vi "Recursive Add Item References to Map.vi"(8 "error in (no error)":errorcluster, 10 "ProjectItem Refnum":refnum<vi>, 11 "Icon Decorator In":refnum<class "Icon Decorator.lvclass">) -> (0 "error out":errorcluster, 3 "Icon Decorator Out":refnum<class "Icon Decorator.lvclass">)   [LabVIEW 2020, in "Icon Decorator.lvclass"]
uses:
  Icon Decorator.lvclass
  LUnit Test Case.lvclass
  Icon Decorator.lvclass/Icon Decorator.ctl
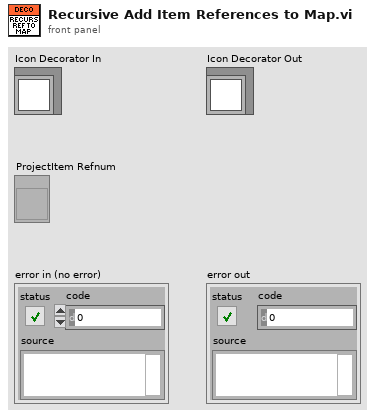
[diagram p1: front panel]
types:
  T1 = typedef "ItemRef.ctl" = u64
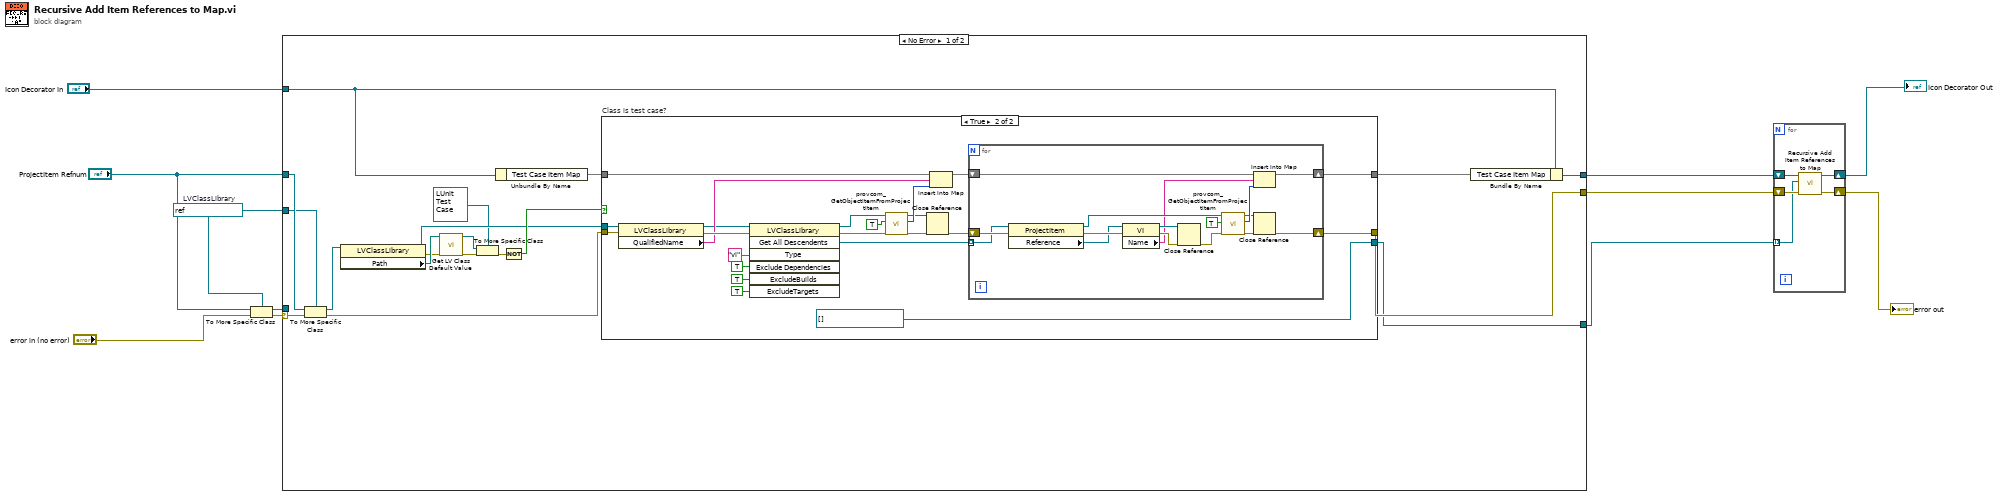
[diagram p0: block diagram]
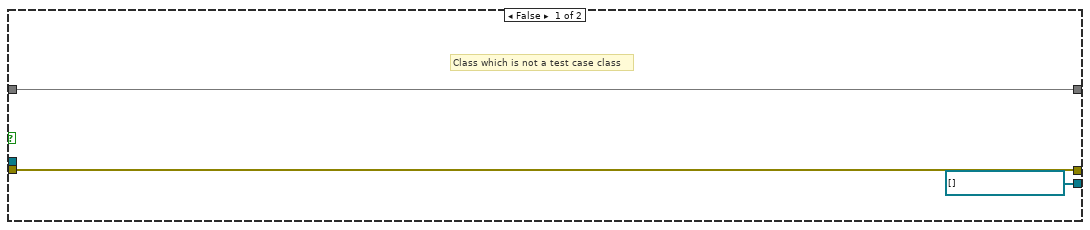
[diagram p2: hidden frame]
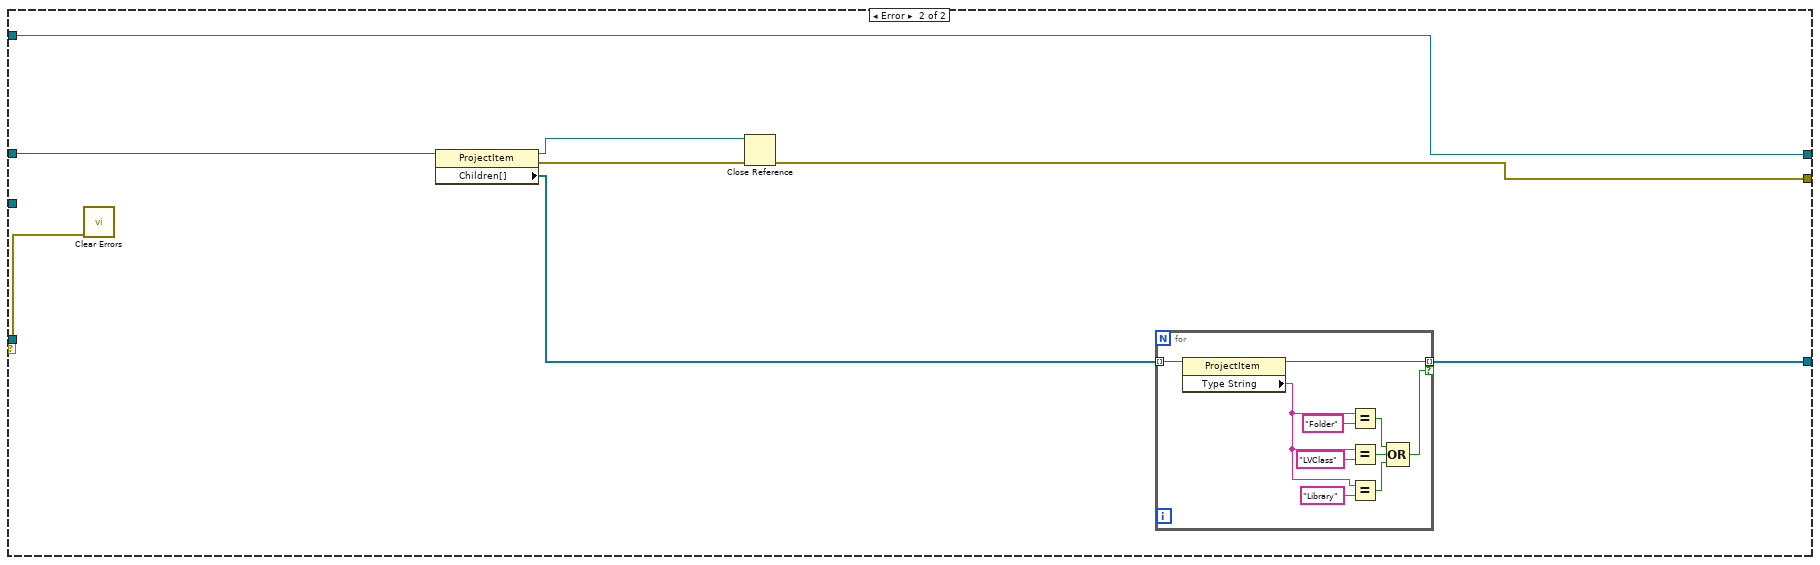
[diagram p3: hidden frame]
diagram:
  w1 = refnum<vi> refnum  # LVClassLibrary
  n1 = To More Specific Class(target class=w1, reference="ProjectItem Refnum", error in="error in (no error)") -> (specific class reference=w3:refnum<vi>, error out=w4:errorcluster)
  n2 = case shown="No Error" w4 {
    selector: w4 -> [w24 w76]
    tunnel: "Icon Decorator In" -> [w30 w74]
    tunnel: [w27 w75] -> w10
    tunnel: [w26 w74] -> w8
    tunnel: [w25 w72] -> w6
    tunnel: w3 -> [_ _]
    tunnel: "ProjectItem Refnum" -> [w22 w77]
    tunnel: w1 -> [w21 _]
    frame No Error {
      n3 = To More Specific Class(target class=w21, reference=w22, error in=w24) -> (specific class reference=w19:refnum<vi>, error out=w23:errorcluster)
      n4 = property class="LVClassLibrary"(reference=w19) -> (reference out=w18:refnum<vi>, error out=w14:errorcluster, "Path"=w15:path)  [unwired: 1 in]
      n5 = call <vilib>:"Get LV Class Default Value.vi"("error in (no error)"=w14, "class path"=w15) -> ("error out"=w12:errorcluster, "object"=w13:refnum<class>)  [unwired: 8 in]
      n6 = To More Specific Class(target class=refnum<class "LUnit Test Case.lvclass"> refnum ("LUnit Test Case V2.lvclass"), reference=w13, error in=w12) -> (error out=w16:errorcluster)  [unwired: 1 out]
      n7 = Unbundle By Name(w30) -> ("Test Case Item Map"=w28:map{string, T1})
      n8 = Not(x=w16) -> (.not. x?=w20:bool)
      n9 = case "Class is test case?" shown="True" w20 {
        tunnel: w28 -> [w33 w54]
        tunnel: w18 -> [_ w53]
        tunnel: w23 -> [w32 w48]
        tunnel: [w32 w38] -> w27
        tunnel: [w33 w40] -> w29
        tunnel: [refnum<vi>[] [] ("Children[]") refnum<vi>[] [] ("Children[]")] -> w25
        frame False {
          # "Class which is not a test case class"
        }
        frame True {
          n10 = property class="LVClassLibrary"(reference=w53, error in=w48) -> (reference out=w43:refnum<vi>, error out=w47:errorcluster, "QualifiedName"=w46:string)
          n11 = invoke class="LVClassLibrary" method="Get All Descendents"(reference=w43, error in=w47, "Type"="vi", "Exclude Dependencies"=TRUE ("ExcludeDependencies"), "ExcludeBuilds"=TRUE, "ExcludeTargets"=TRUE) -> (reference out=w42:refnum<vi>, error out=w44:errorcluster, "All Descendents"=w37:refnum<vi>[])  [unwired: 1 in, 4 out]
          n12 = call <resource>:"provcom_GetObjectItemFromProjectItem.vi"("error in (no error)"=w44, "bind? (Y)"=TRUE, "ProjectItem"=w42) -> ("error out"=w50:errorcluster, "ObjectItem"=w52:T1, "dup ProjectItem"=w51:refnum<vi>)  [unwired: 6 in]
          n13 = Close Reference(reference=w51, error in (no error)=w50) -> (error out=w39:errorcluster)
          n14 = Insert Into Map(map in=w54, key=w46, value=w52) -> (map out=w49:map{string, T1})  [unwired: 2 out]
          n15 = for {
            tunnel: w37 -> [w67] mode=indexing
            shift-right: [w70] -> w40
            shift-left: w49 -> [w71]
            shift-right: [w65] -> w38
            shift-left: w39 -> [w69]
            n16 = property class="ProjectItem"(reference=w67, error in=w69) -> (reference out=w66:refnum<vi>, error out=w68:errorcluster, "Reference"=w64:refnum<vi>)
            n17 = property class="VI"(reference=w64, error in=w68) -> (reference out=w57:refnum<vi>, error out=w59:errorcluster, "Name"=w56:string)
            n18 = Close Reference(reference=w57, error in (no error)=w59) -> (error out=w58:errorcluster)
            n19 = call <resource>:"provcom_GetObjectItemFromProjectItem.vi"("error in (no error)"=w58, "bind? (Y)"=TRUE, "ProjectItem"=w66) -> ("error out"=w62:errorcluster, "ObjectItem"=w63:T1, "dup ProjectItem"=w61:refnum<vi>)  [unwired: 6 in]
            n20 = Insert Into Map(map in=w71, key=w56, value=w63) -> (map out=w70:map{string, T1})  [unwired: 2 out]
            n21 = Close Reference(reference=w61, error in (no error)=w62) -> (error out=w65:errorcluster)
          }
        }
      }
      n22 = Bundle By Name(cluster=w30, "Test Case Item Map"=w29) -> (w26:refnum<class "Icon Decorator.lvclass">)
    }
    frame Error {
      n23 = call <vilib>:"Clear Errors.vi"("error in (no error)"=w76) -> ()  [unwired: 5 in, 2 out]
      n24 = property class="ProjectItem"(reference=w77) -> (reference out=w79:refnum<vi>, error out=w78:errorcluster, "Children[]"=w73:refnum<vi>[])  [unwired: 1 in]
      n25 = Close Reference(reference=w79, error in (no error)=w78) -> (error out=w75:errorcluster)
      n26 = for {
        tunnel: w73 -> [w89] mode=indexing
        tunnel: [w87] -> w72 mode=indexing if=w84
        n27 = property class="ProjectItem"(reference=w89) -> (reference out=w87:refnum<vi>, "Type String"=w81:string)  [unwired: 1 in, 1 out]
        n28 = Equal?(x=w81, y="Folder") -> (x = y?=w85:bool)
        n29 = Equal?(x=w81, y="LVClass") -> (x = y?=w83:bool)
        n30 = Equal?(x=w81, y="Library" ("Type")) -> (x = y?=w80:bool)
        n31 = Compound Arithmetic op=OR(w85, w83, w80) -> (w84:bool)
      }
    }
  }
  n32 = for {
    shift-right: [w93] -> w9
    shift-left: w10 -> [w94]
    shift-right: [w91] -> w7
    shift-left: w8 -> [w92]
    tunnel: w6 -> [w90] mode=indexing
    n33 = call "Recursive Add Item References to Map.vi"("error in (no error)"=w94, "ProjectItem Refnum"=w90, "Icon Decorator In"=w92) -> ("error out"=w93:errorcluster, "Icon Decorator Out"=w91:refnum<class "Icon Decorator.lvclass">)  [unwired: 7 in]
  }
  "Icon Decorator Out" <- w7
  "error out" <- w9
